vi "Open Drive.vi"(8 "error in (no error)":errorcluster) -> (0 "error out":errorcluster)   [LabVIEW 2018]
uses:
  TypeDefs/typedef_enum_Refnums.ctl
  <vilib>/Rock Robotics/WPI/ThirdParty/Phoenix-LabVIEW/Motor Controller/Controls/CTRE_Phoenix_MotorControl_NeutralMode.ctl
  <vilib>/Rock Robotics/WPI/RobotDrive/WPI_RobotDriveOpen2MotorWithExistingMotors.vi
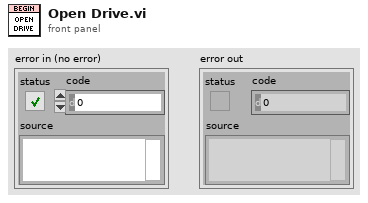
[diagram p1: front panel]
types:
  T1 = typedef "CTRE_Phoenix_MotorControl_NeutralMode.ctl" = enum8{"EEPROMSetting", "Override to Coast", "Override to Brake"}
  T2 = typedef "typedef_enum_Refnums.ctl" = enum16{"Ball_Encoder", "Ball_Motor", "Camera", "Linefollow_3", "Linefollow_2", "Linefollow_1", "Gyro", "Hatch_Solenoid", "Climb_Back_Solenoid", "Arm_Encoder", "Arm_Motor", "Lift_Encoder", "Drive", "Drive_Motor_R", "Drive_Motor_L", "Drive_Encoder_R", "Drive_Encoder_L", "Joy_R", "Joy_L", "Wrist_Motor", "Wrist_Encoder", "Climb Upper Limit", "Climb Lower Limit ", "Climb_Front_Motor"}
  T3 = typedef "WPI_MotorControlDeviceRef.ctl" = cluster{"DeviceStatus":errorcluster, "Type":T4, "PWM":cluster{"PWM Channel":T5, "DeadBand":T6}, "CAN":cluster{"Device Number":u8, "SetOutput VI Ref":variant, "GetOutput VI Ref":variant, "Enable VI Ref":variant, "Disable VI Ref":variant, "Data":variant}, "Invert":bool, "DIO PWM":cluster{"PWM \"Enable\" Channel":T5, "DIOChannel":T7, "PWM Rate":dbl}}
  T4 = typedef "WPI_MotorControlType.ctl" = enum16{"PWM", "CAN", "DIO PWM"}
  T5 = typedef "FPGA_DIOPWMChannel.ctl" = enum8{"PWM 0", "PWM 1", "PWM 2", "PWM 3", "PWM 4", "PWM 5", "PWM 6", "PWM 7", "PWM 8", "PWM 9", "PWM MXP 0", "PWM MXP 1", "PWM MXP 2", "PWM MXP 3", "PWM MXP 4", "PWM MXP 5", "PWM MXP 6", "PWM MXP 7", "PWM MXP 8", "PWM MXP 9", "Invalid"}
  T6 = typedef "WPI_PWMDeadband.ctl" = cluster{"Name":string, "maxPositivePwm":i32, "minPositivePwm":i32, "centerPwm":i32, "maxNegativePwm":i32, "minNegativePwm":i32, "angularRange":u16}
  T7 = typedef "FPGA_DIOChannel.ctl" = enum8{"DIO 0", "DIO 1", "DIO 2", "DIO 3", "DIO 4", "DIO 5", "DIO 6", "DIO 7", "DIO 8", "DIO 9", "DIO MXP 0", "DIO MXP 1", "DIO MXP 2", "DIO MXP 3", "DIO MXP 4", "DIO MXP 5", "DIO MXP 6", "DIO MXP 7", "DIO MXP 8", "DIO MXP 9", "DIO MXP 10", "DIO MXP 11", "DIO MXP 12", "DIO MXP 13", "DIO MXP 14", "DIO MXP 15", "SPI Port CS1", "SPI Port CS2", "SPI Port CS3", "SPI Port MISO", "SPI Port MOSI", "Invalid"}
  T8 = typedef "WPI_RobotDriveDevRef.ctl" = cluster{"DevStatus":errorcluster, "Motors[]":T3[], "Square Inputs":bool, "Max Output":dbl}
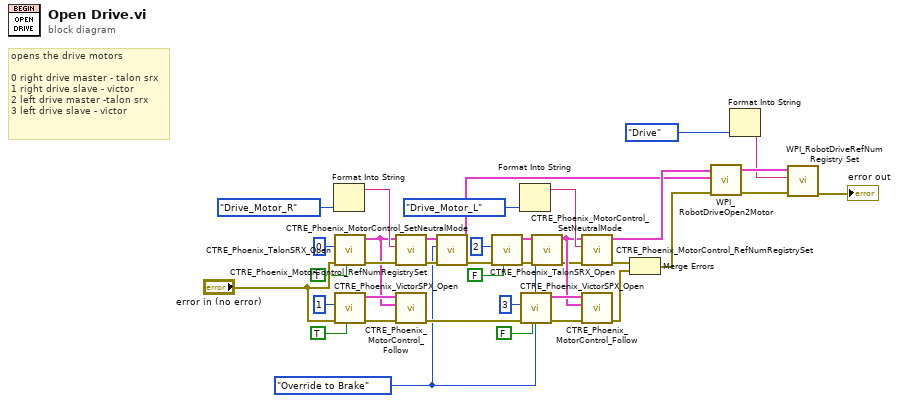
[diagram p0: block diagram]
diagram:
  w1 = CTRE_Phoenix_MotorControl_NeutralMode."Override to Brake" ("Motor Control Neutral Mode")
  # "opens the drive motors \n\n0 right drive master - talon srx\n1 right drive slave - victor\n2 left drive master -talon srx\n3 left drive slave - victor"
  n1 = Format Into String(typedef_enum_Refnums."Drive_Motor_R" ("RefNums")) -> (resulting string=w36:string)  [unwired: 3 in, 1 out]
  n2 = call <vilib>:"CTRE_Phoenix_TalonSRX_Open.vi"("Invert"=TRUE, "error in"="error in (no error)", "Device Number"=u8 0) -> ("error out"=w38:errorcluster, "CAN Talon SRX Ref"=w32:T3)  [unwired: 7 in]
  n3 = call <vilib>:"CTRE_Phoenix_VictorSPX_Open.vi"("Invert"=TRUE, "error in"="error in (no error)", "Device Number"=u8 1) -> ("error out"=w34:errorcluster, "CAN Talon SRX Ref"=w33:T3)  [unwired: 7 in]
  n4 = call <vilib>:"CTRE_Phoenix_MotorControl_RefNumRegistrySet.vi"("error in (no error)"=w38, "refnum name"=w36, "PhoenixMotorControlDevRef"=w32) -> ("error out"=w6:errorcluster, "PhoenixMotorControlDevRef"=w11:T3)  [unwired: 7 in]
  n5 = call <vilib>:"CTRE_Phoenix_MotorControl_Follow.vi"("error in (no error)"=w34, "Master Controller to Follow"=w32, "PhoenixMotorControlDevRef"=w33) -> ("error out"=w19:errorcluster)  [unwired: 7 in, 1 out]
  n6 = call <vilib>:"CTRE_Phoenix_MotorControl_SetNeutralMode.vi"("error in (no error)"=w6, "Motor Control Neutral Mode"=w1, "PhoenixMotorControlDevRef"=w11) -> ("error out"=w5:errorcluster, "PhoenixMotorControlDevRef"=w7:T3)  [unwired: 7 in]
  n7 = call <vilib>:"CTRE_Phoenix_TalonSRX_Open.vi"("Invert"=FALSE, "error in"=w5, "Device Number"=u8 2) -> ("error out"=w3:errorcluster, "CAN Talon SRX Ref"=w29:T3)  [unwired: 7 in]
  n8 = Format Into String(typedef_enum_Refnums."Drive_Motor_L" ("RefNums")) -> (resulting string=w25:string)  [unwired: 3 in, 1 out]
  n9 = call <vilib>:"CTRE_Phoenix_VictorSPX_Open.vi"("Invert"=FALSE, "error in"=w19, "Device Number"=u8 3) -> ("error out"=w27:errorcluster, "CAN Talon SRX Ref"=w28:T3)  [unwired: 7 in]
  n10 = call <vilib>:"CTRE_Phoenix_MotorControl_SetNeutralMode.vi"("error in (no error)"=w3, "Motor Control Neutral Mode"=w1, "PhoenixMotorControlDevRef"=w29) -> ("error out"=w2:errorcluster, "PhoenixMotorControlDevRef"=w4:T3)  [unwired: 7 in]
  n11 = call <vilib>:"CTRE_Phoenix_MotorControl_RefNumRegistrySet.vi"("error in (no error)"=w2, "refnum name"=w25, "PhoenixMotorControlDevRef"=w4) -> ("error out"=w17:errorcluster, "PhoenixMotorControlDevRef"=w10:T3)  [unwired: 7 in]
  n12 = call <vilib>:"CTRE_Phoenix_MotorControl_Follow.vi"("error in (no error)"=w27, "Master Controller to Follow"=w4, "PhoenixMotorControlDevRef"=w28) -> ("error out"=w18:errorcluster)  [unwired: 7 in, 1 out]
  n13 = Merge Errors(w17, w18) -> (w16:errorcluster)
  n14 = call-poly <vilib>:"WPI_RobotDriveOpen2Motor.vi"("error in (no error)"=w16, "Right Motor Dev Ref"=w7, "Left Motor Dev Ref"=w10) -> ("error out"=w22:errorcluster, "RobotDriveDevRef"=w23:T8)  [unwired: 7 in]
  n15 = Format Into String(typedef_enum_Refnums."Drive" ("RefNums")) -> (resulting string=w8:string)  [unwired: 3 in, 1 out]
  n16 = call <vilib>:"WPI_RobotDriveRefNum Registry Set.vi"("error in (no error)"=w22, "refnum name"=w8, "RobotDriveDevRef"=w23) -> ("error out"=→"error out":errorcluster)  [unwired: 7 in, 1 out]
